vi "TDMS.GetAnalysisResults.vi"(8 "error in (no error)":errorcluster, 11 "Refnum in":refnum<k34>) -> (0 "error out":errorcluster, 2 "Variant":variant, 3 "Refnum out":refnum<k34>)   [LabVIEW 2015, in "NIAnalysis.lvlib"]
uses:
  NIAnalysis.lvlib
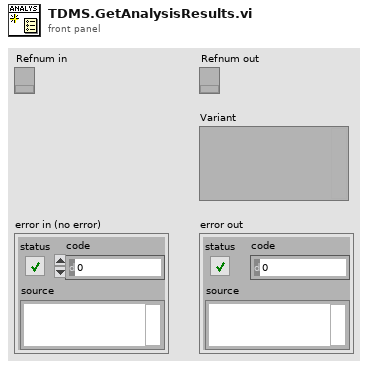
[diagram p1: front panel]
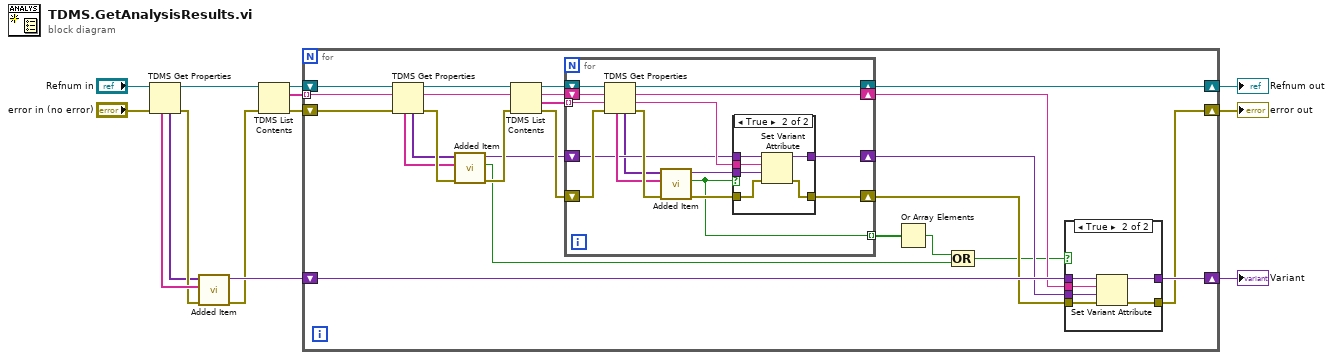
[diagram p0: block diagram]
diagram:
  n1 = TDMS Get Properties(8:"error in (no error)", 11:"Refnum in") -> (0:w3:errorcluster, 3:w6:refnum<k34>, 4:w1:variant[], 6:w4:string[])  [unwired: 4 in, 2 out]
  n2 = call "Added Item.vi"("error in (no error)"=w3, "property names"=w4, "property values"=w1) -> ("error out"=w2:errorcluster, "Variant out"=w5:variant)  [unwired: 6 in, 1 out]
  n3 = TDMS List Contents(4:w2, 7:w6) -> (0:w13:errorcluster, 2:w9:string[], 3:w10:refnum<k34>)  [unwired: 1 in, 1 out]
  n4 = for {
    tunnel: w9 -> [w31] mode=indexing
    shift-right: [w24] -> w11
    shift-left: w13 -> [w34]
    shift-right: [w39] -> w12
    shift-left: w10 -> [w33]
    shift-right: [w25] -> w14
    shift-left: w5 -> [w27]
    n5 = TDMS Get Properties(8:w34, 10:w31, 11:w33) -> (0:w29:errorcluster, 2:w30:string, 3:w32:refnum<k34>, 4:w19:variant[], 6:w28:string[])  [unwired: 3 in, 1 out]
    n6 = call "Added Item.vi"("error in (no error)"=w29, "property names"=w28, "property values"=w19) -> ("error out"=w26:errorcluster, "Result?"=w16:bool, "Variant out"=w23:variant)  [unwired: 6 in]
    n7 = TDMS List Contents(4:w26, 6:w30, 7:w32) -> (0:w38:errorcluster, 1:w35:string[], 2:w36:string, 3:w37:refnum<k34>)
    n8 = for {
      tunnel: w35 -> [w63] mode=indexing
      shift-right: [w54] -> w21
      shift-left: w38 -> [w61]
      shift-right: [w59] -> w39
      shift-left: w37 -> [w60]
      shift-right: [w56] -> w20
      shift-left: w36 -> [w62]
      shift-right: [w50] -> w22
      shift-left: w23 -> [w51]
      tunnel: [w48] -> w18 mode=indexing
      n9 = TDMS Get Properties(8:w61, 9:w63, 10:w62, 11:w60) -> (0:w58:errorcluster, 1:w52:string, 2:w56:string, 3:w59:refnum<k34>, 4:w49:variant[], 6:w57:string[])  [unwired: 2 in]
      n10 = call "Added Item.vi"("error in (no error)"=w58, "property names"=w57, "property values"=w49) -> ("error out"=w55:errorcluster, "Result?"=w48:bool, "Variant out"=w53:variant)  [unwired: 6 in]
      n11 = case shown="True" w48 {
        tunnel: w55 -> [w64 w71]
        tunnel: [w64 w70] -> w54
        tunnel: w53 -> [_ w69]
        tunnel: w52 -> [_ w68]
        tunnel: w51 -> [w65 w67]
        tunnel: [w65 w66] -> w50
        frame False {
        }
        frame True {
          n12 = Set Variant Attribute(Variant=w67, name=w68, value=w69, error in=w71) -> (Variant out=w66:variant, error out=w70:errorcluster)  [unwired: 1 out]
        }
      }
    }
    n13 = Or Array Elements(Boolean array=w18) -> (logical OR=w17:bool)
    n14 = Compound Arithmetic op=OR(w17, w16) -> (w15:bool)
    n15 = case shown="True" w15 {
      tunnel: w27 -> [w40 w47]
      tunnel: [w40 w46] -> w25
      tunnel: [w41 w45] -> w24
      tunnel: w22 -> [_ w44]
      tunnel: w21 -> [w41 w43]
      tunnel: w20 -> [_ w42]
      frame False {
      }
      frame True {
        n16 = Set Variant Attribute(Variant=w47, name=w42, value=w44, error in=w43) -> (Variant out=w46:variant, error out=w45:errorcluster)  [unwired: 1 out]
      }
    }
  }
  "Variant" <- w14
  "Refnum out" <- w12
  "error out" <- w11
